vi "Panel Resized.vi"(6 "Sizing Refnums":T2, 8 "error in (no error)":errorcluster, 9 "Origin":cluster{"H":i16, "V":i16}, 10 "NewBnds":T1, 11 "Size Constraints":cluster{"min tab width":i32, "w/h":dbl}) -> (0 "error out":errorcluster)   [LabVIEW 2016]
uses:
  <vilib>/Utility/miscctls.llb/LVRectTypeDef.ctl
  <vilib>/Utility/miscctls.llb/LVRowAndColumnTypeDef.ctl
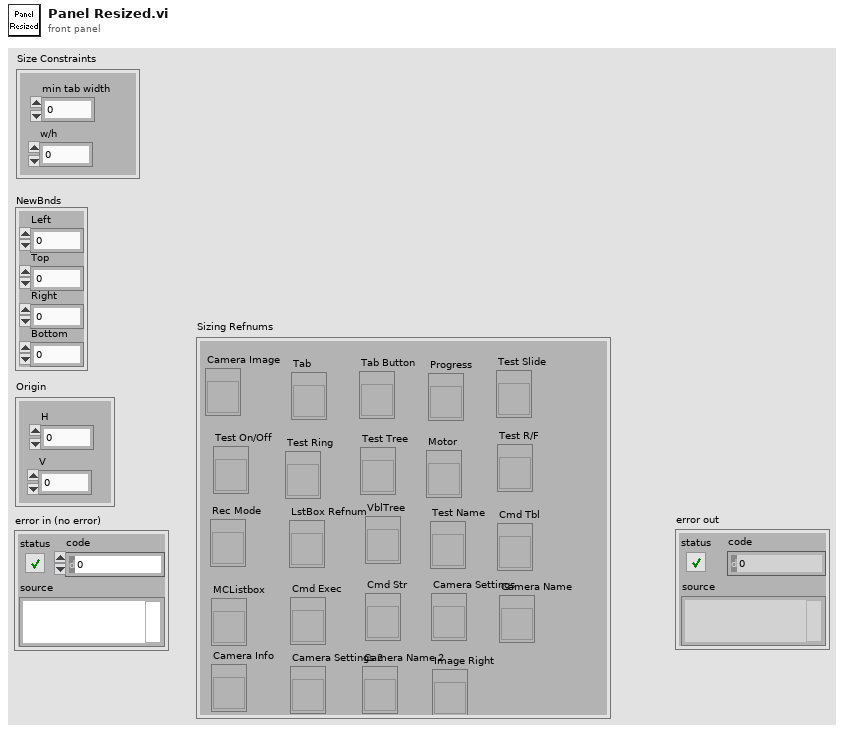
[diagram p1: front panel]
types:
  T1 = typedef "LVRectTypeDef.ctl" = cluster{"Left":i16, "Top":i16, "Right":i16, "Bottom":i16}
  T2 = cluster{"Camera Image":refnum<vi>, "Tab":refnum<vi>, "Tab Button":refnum<vi>, "Rec Mode":refnum<vi>, "Test Slide":refnum<vi>, "Test On/Off":refnum<vi>, "Test Ring":refnum<vi>, "Test R/F":refnum<vi>, "Test Name":refnum<vi>, "Motor":refnum<vi>, "Progress":refnum<vi>, "LstBox Refnum":refnum<vi>, "Test Tree":refnum<vi>, "VblTree":refnum<vi>, "Cmd Tbl":refnum<vi>, "MCListbox":refnum<vi>, "Cmd Exec":refnum<vi>, "Cmd Str":refnum<vi>, "Camera Settings":refnum<vi>, "Camera Name":refnum<vi>, "Camera Info":refnum<vi>, "Camera Settings 2":refnum<vi>, "Camera Name 2":refnum<vi>, "Image Right":refnum<vi>}
  T3 = typedef "LVRowAndColumnTypeDef.ctl" = cluster{"Row":i32, "Column":i32}
  T4 = typedef "LVPositionTypeDef.ctl" = cluster{"Left":i32, "Top":i32}
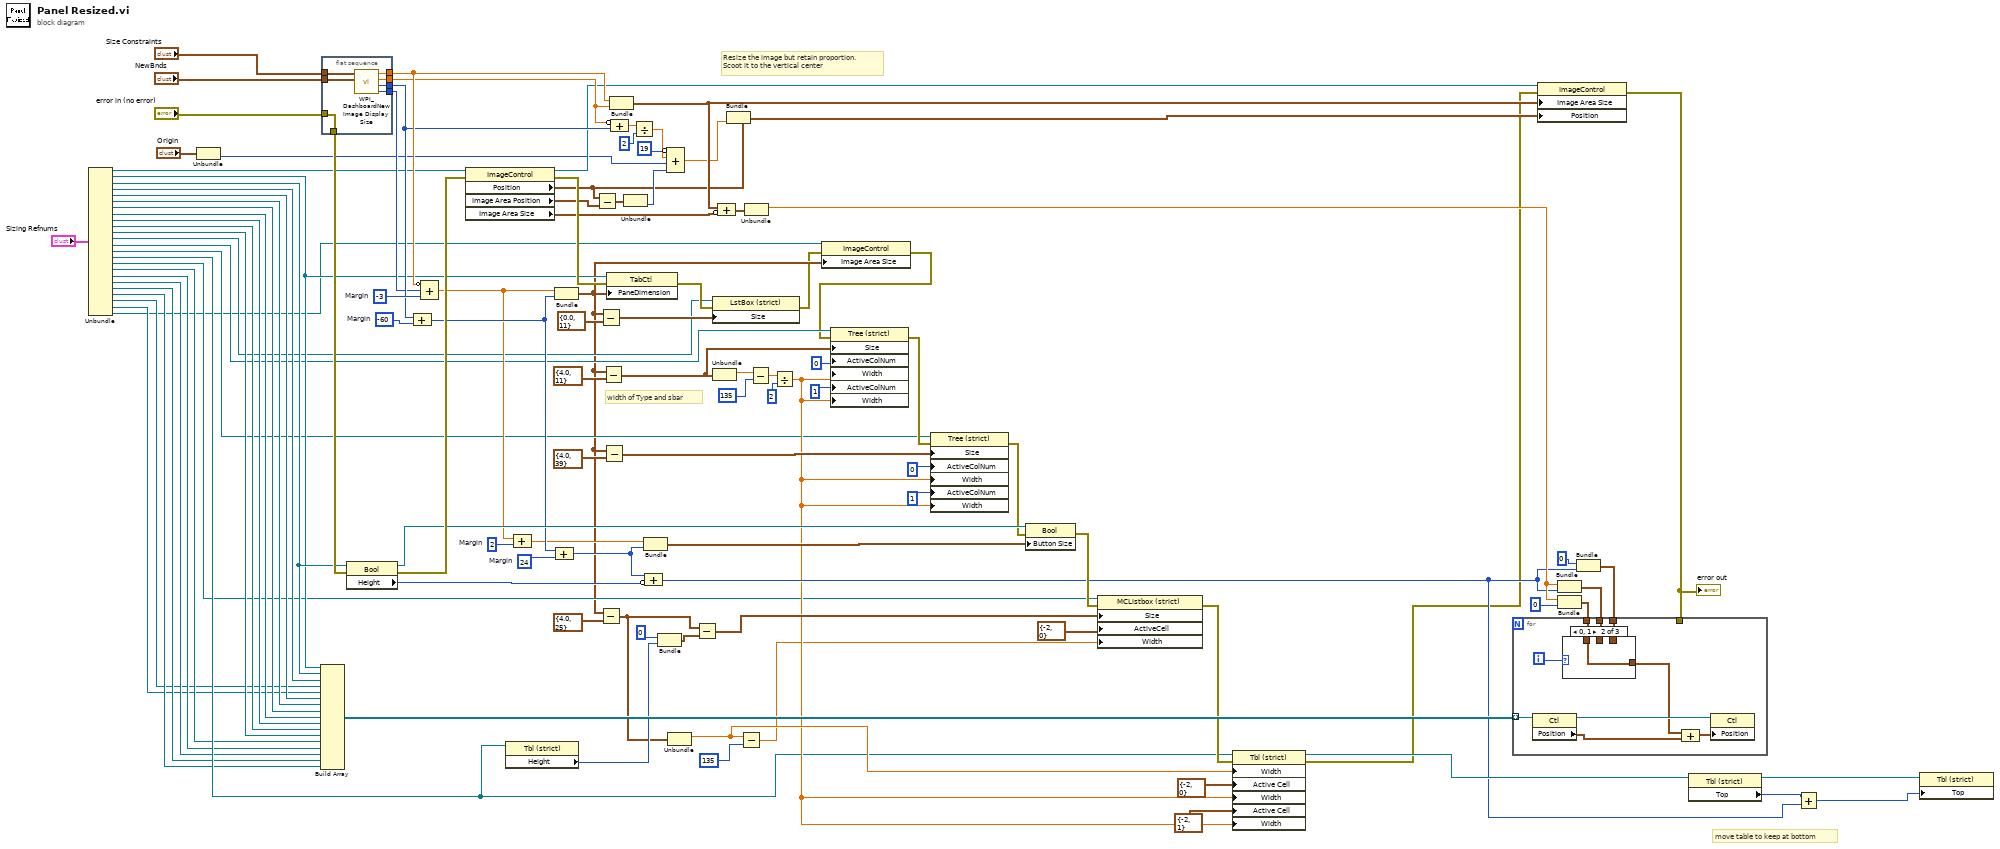
[diagram p0: block diagram]
diagram:
  w98 = 24  # Margin
  w96 = 2  # Margin
  w92 = -60  # Margin
  w102 = -3  # Margin
  # "move table to keep at bottom"
  # "width of Type and sbar"
  # "Resize the image but retain proportion.\nScoot it to the vertical center"
  n1 = Unbundle("Sizing Refnums") -> ("Camera Image"=w67:refnum<vi>, "Tab"=w68:refnum<vi>, "Tab Button"=w75:refnum<vi>, "Rec Mode"=w26:refnum<vi>, "Test Slide"=w25:refnum<vi>, "Test On/Off"=w24:refnum<vi>, "Test Ring"=w23:refnum<vi>, "Test R/F"=w22:refnum<vi>, "Test Name"=w21:refnum<vi>, "Motor"=w20:refnum<vi>, "Progress"=w19:refnum<vi>, "LstBox Refnum"=w18:refnum<vi>, "Test Tree"=w17:refnum<vi>, "VblTree"=w16:refnum<vi>, "Cmd Tbl"=w15:refnum<vi>, "MCListbox"=w14:refnum<vi>, "Cmd Exec"=w13:refnum<vi>, "Cmd Str"=w12:refnum<vi>, "Camera Settings"=w11:refnum<vi>, "Camera Name"=w10:refnum<vi>, "Camera Info"=w9:refnum<vi>, "Camera Settings 2"=w8:refnum<vi>, "Camera Name 2"=w7:refnum<vi>, "Image Right"=w3:refnum<vi>)
  n2 = Unbundle("Origin") -> ("V"=w72:i16)  [unwired: 1 out]
  n3 = Build Array(w68, w75, w26, w8, w7, w25, w24, w23, w22, w21, w20, w19, w13, w12, w11, w10, w9) -> (w111:refnum<vi>[])
  n4 = flat-sequence {
    tunnel: "NewBnds" -> [w118]
    tunnel: "Size Constraints" -> [w117]
    tunnel: [w116] -> w91
    tunnel: [w115] -> w99
    tunnel: [w114] -> w100
    tunnel: [w113] -> w101
    tunnel: [w112] -> w110
    tunnel: "error in (no error)" -> [w112]
    frame #0 {
      n5 = call <vilib>:"WPI_DashboardNew Image Display Size.vi"("NewBnds"=w118, "Size Constraints"=w117) -> ("Window Width"=w116:i16, "Window Height"=w114:i16, "Height"=w115:dbl, "Width"=w113:dbl)  [unwired: 6 in]
    }
  }
  n6 = property class="Bool"(reference=w75, error in=w110) -> (reference out=w105:refnum<vi>, error out=w109:errorcluster, "Height"=w104:u32)
  n7 = Compound Arithmetic op=unknown(w100, w92) -> (w97:i32)
  n8 = Compound Arithmetic op=ADD(invert w101, w91, w102) -> (w95:dbl)
  n9 = property class="ImageControl"(reference=w67, error in=w109) -> (reference out=w84:refnum<vi>, error out=w108:errorcluster, "Position"=w83:T4, "Image Area Position"=w78:cluster{"Left":i32, "Top":i32}, "Image Area Size"=w89:cluster{"Width":u32, "Height":u32})
  n10 = property class="Tbl (strict)"(reference=w15) -> ("Height"=w43:u32)  [unwired: 1 in, 2 out]
  n11 = Compound Arithmetic op=ADD(w95, w96) -> (w94:dbl)
  n12 = Bundle(w95, w97) -> (w6:cluster{dbl, i32})  [unwired: 1 in]
  n13 = Compound Arithmetic op=ADD(w97, w98) -> (w103:i32)
  n14 = Subtract(x=w83, y=w78) -> (x-y=w85:T4)
  n15 = Subtract(x=w6, y=cluster{dbl, i32} {0.0, 11}) -> (x-y=w65:cluster{dbl, i32})
  n16 = Subtract(x=w6, y=cluster{dbl, i32} {4.0, 25}) -> (x-y=w40:cluster{dbl, i32})
  n17 = Subtract(x=w6, y=cluster{dbl, i32} {4.0, 11}) -> (x-y=w56:cluster{dbl, i32})
  n18 = Subtract(x=w6, y=cluster{dbl, i32} {4.0, 39}) -> (x-y=w61:cluster{dbl, i32})
  n19 = property class="TabCtl"(reference=w68, error in=w108, "PaneDimension"=w6) -> (error out=w66:errorcluster)  [unwired: 1 out]
  n20 = Bundle("Width"=w101, "Height"=w99) -> (w87:cluster{"Width":dbl, "Height":dbl})  [unwired: 1 in]
  n21 = Compound Arithmetic op=ADD(invert w99, w100) -> (w79:dbl)
  n22 = Unbundle(w85) -> ("Top"=w86:i32)  [unwired: 1 out]
  n23 = Divide(x=w79, y=2) -> (x/y=w81:dbl)
  n24 = Bundle(w94, w103) -> (w93:cluster{dbl, i32})  [unwired: 1 in]
  n25 = Compound Arithmetic op=ADD(w103, invert w104) -> (w35:u32)
  n26 = Bundle(0, "Height"=w43) -> (w41:cluster{i32, "Height":u32})  [unwired: 1 in]
  n27 = Compound Arithmetic op=ADD(invert 19, w81, w72, w86) -> (w82:dbl)
  n28 = Unbundle(w40) -> (w31:dbl)  [unwired: 1 out]
  n29 = Subtract(x=w40, y=w41) -> (x-y=w39:cluster{dbl, u32})
  n30 = property class="LstBox (strict)"(reference=w18, error in=w66, "Size"=w65) -> (error out=w5:errorcluster)  [unwired: 1 out]
  n31 = Unbundle(w56) -> (w55:dbl)  [unwired: 1 out]
  n32 = Compound Arithmetic op=ADD(w87, invert w89) -> (w90:cluster{"Width":dbl, "Height":dbl})
  n33 = Bundle(cluster=w83, "Top"=w82) -> (w88:T4)  [unwired: 1 in]
  n34 = Subtract(x=w31, y=135) -> (x-y=w28:dbl)
  n35 = Unbundle(w90) -> ("Width"=w106:dbl)  [unwired: 1 out]
  n36 = Subtract(x=w55, y=135 ("Active Cell:Active Column Number")) -> (x-y=w51:dbl)
  n37 = Divide(x=w51, y=2 ("Active Cell:Active Column Number")) -> (x/y=w29:dbl)
  n38 = property class="ImageControl"(reference=w3, error in=w5, "Image Area Size"=w6) -> (error out=w4:errorcluster)  [unwired: 1 out]
  n39 = property class="Tree (strict)"(reference=w17, error in=w4, "Size"=w56, "ActiveColNum"=0 ("Active Cell:Active Column Number"), "Width"=w29, "ActiveColNum"=1 ("Active Cell:Active Column Number"), "Width"=w29) -> (error out=w60:errorcluster)  [unwired: 1 out]
  n40 = property class="Tree (strict)"(reference=w16, error in=w60, "Size"=w61, "ActiveColNum"=0 ("Active Cell:Active Column Number"), "Width"=w29, "ActiveColNum"=1 ("Active Cell:Active Column Number"), "Width"=w29) -> (error out=w59:errorcluster)  [unwired: 1 out]
  n41 = property class="Bool"(reference=w105, error in=w59, "Button Size"=w93) -> (error out=w47:errorcluster)  [unwired: 1 out]
  n42 = property class="MCListbox (strict)"(reference=w14, error in=w47, "Size"=w39, "ActiveCell"=T3 {"Row"=-2, "Column"=0} ("Active Cell:Active Cell"), "Width"=w28) -> (error out=w44:errorcluster)  [unwired: 1 out]
  n43 = property class="Tbl (strict)"(reference=w15, error in=w44, "Width"=w31, "Active Cell"=T3 {"Row"=-2, "Column"=0} ("Active Cell:Active Cell"), "Width"=w29, "Active Cell"=T3 {"Row"=-2, "Column"=1} ("Active Cell:Active Cell"), "Width"=w29) -> (reference out=w38:refnum<vi>, error out=w2:errorcluster)
  n44 = property class="ImageControl"(reference=w84, error in=w2, "Image Area Size"=w87, "Position"=w88) -> (error out=w1:errorcluster)  [unwired: 1 out]
  "error out" <- w1
  n45 = Bundle("Width"=w106, w35) -> (w77:cluster{"Width":dbl, u32})  [unwired: 1 in]
  n46 = Bundle("Width"=w106, 0) -> (w76:cluster{"Width":dbl, i32})  [unwired: 1 in]
  n47 = Bundle(0, w35) -> (w48:cluster{i32, u32})  [unwired: 1 in]
  n48 = for {
    tunnel: w111 -> [w127] mode=indexing
    tunnel: w77 -> [w121]
    tunnel: w76 -> [w122]
    tunnel: w1 -> [_]
    tunnel: w48 -> [w120]
    i -> [w123]
    n49 = property class="Ctl"(reference=w127) -> (reference out=w126:refnum<vi>, "Position"=w125:T4)  [unwired: 1 in, 1 out]
    n50 = case shown="0, 1" w123 {
      tunnel: w122 -> [_ w129 _]
      tunnel: w121 -> [_ _ w130]
      tunnel: w120 -> [w128 _ _]
      tunnel: [w128 w129 w130] -> w119
      frame Default {
      }
      frame 0, 1 {
      }
      frame 2..4 {
      }
    }
    n51 = Compound Arithmetic op=ADD(w119, w125) -> (w124:cluster{dbl, u32})
    n52 = property class="Ctl"(reference=w126, "Position"=w124) -> ()  [unwired: 1 in, 2 out]
  }
  n53 = property class="Tbl (strict)"(reference=w38) -> (reference out=w37:refnum<vi>, "Top"=w36:i32)  [unwired: 1 in, 1 out]
  n54 = Add(x=w36, y=w35) -> (x+y=w34:u32)
  n55 = property class="Tbl (strict)"(reference=w37, "Top"=w34) -> ()  [unwired: 1 in, 2 out]
